vi "ief initialize_example.vi"() -> ()   [LabVIEW 2015, in "IEF Werner.lvlib"]
doc: "The VI is an easy initialize example that demonstrates the use of the basic VIs needed for a successful initilization.\n\nAttention:\nIt is neccessary to set one output - the external stop - to true. Otherwise it is not possible to start online control."
uses:
  IEF Werner.lvlib
panel:
  in  "Axis Number":u16=1 min=1 max=16
  out "error out (no error)":errorcluster
  out "Tagprefix out":refnum<k21>
  in  "error in (no error)":errorcluster
  in  "Tagprefix in":refnum<k21>
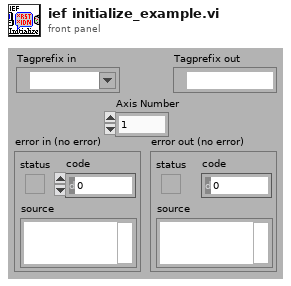
[diagram p1: front panel]
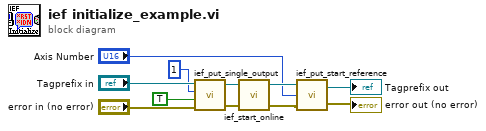
[diagram p0: block diagram]
diagram:
  n1 = call "ief_put_single_output.vi"("error in (no error)"="error in (no error)", "Single Output State"=TRUE, "Single Output Number"=u16 1, "Tagprefix in"="Tagprefix in") -> ("error out (no error)"=w10:errorcluster, "Tagprefix out"=w11:refnum<k21>)  [unwired: 1 out]
  n2 = call "ief_start_online.vi"("Tagprefix in"=w11, "error in (no error)"=w10) -> ("Tagprefix out"=w5:refnum<k21>, "error out (no error)"=w6:errorcluster)  [unwired: 1 out]
  n3 = call "ief_put_start_reference.vi"("error in (no error)"=w6, "Axis Number"="Axis Number", "Tagprefix in"=w5) -> ("error out (no error)"=→"error out (no error)":errorcluster, "Tagprefix out"=→"Tagprefix out":refnum<k21>)
